vi "AcquireDataRamp.vi"(6 "error in":errorcluster, 11 "FPGA VI Reference In":T1) -> (2 "Elements Remaining":u32, 3 "FPGA VI Reference Out":T1, 4 "error out":errorcluster)   [LabVIEW 2016]
uses:
  controls/FPGAVIreferenceTypeDef.ctl
  controls/Enum.ctl
  <vilib>/Utility/error.llb/Error Cluster From Error Code.vi
  <vilib>/rvi/errors/niLvFpgaAdjustHostInterfaceError.vi
  <vilib>/rvi/interface/nirviMethod/nirviMethod.xnode
  FPGA Bitfiles/qnmController797_usbRIO_controllerFPGAmu_11012018-14h.lvbitx
  <vilib>/rvi/errors/niLvFpgaMergeErrorWithErrorCode.vi
  <vilib>/FPGAPlugInAG/USB-7856R OEM/niLvFpga_ReadFifo_USB-7856R OEM.vi
panel:
  # "Enable Error Handling disbaled (from VI properties)"
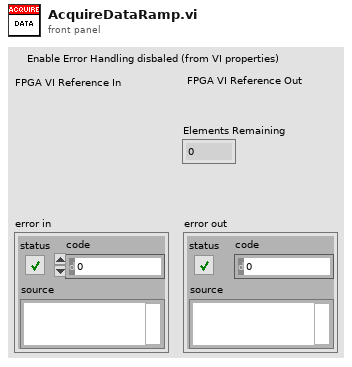
[diagram p1: front panel]
types:
  T1 = typedef "FPGAVIreferenceTypeDef.ctl" = refnum<k20>
  T2 = typedef "Enum.ctl" = enum16{"Init", "Read", "Write"}
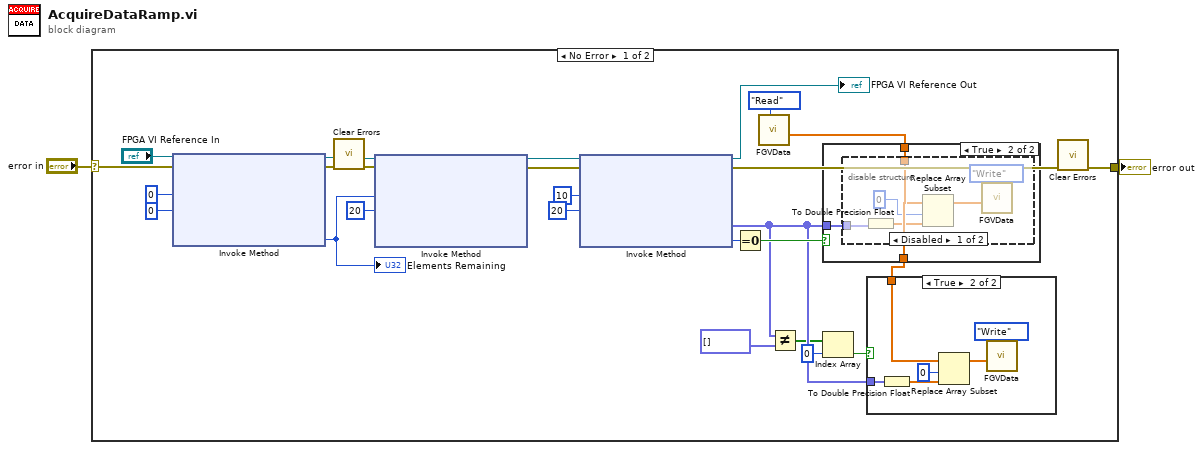
[diagram p0: block diagram]
diagram:
  n1 = case shown="No Error" "error in" {
    selector: "error in" -> [w16 w44]
    tunnel: [w22 w44] -> w2
    frame No Error {
      n2 = xnode "Invoke Method"("FPGA VI Reference In"="FPGA VI Reference In", "error in"=w16, "Number of Elements"=u32 0, "Timeout (ms)"=0) -> ("FPGA VI Reference Out"=w26:T1, "error out"=w28:errorcluster, "Elements Remaining"=w24:u32)  [unwired: 1 out]
      "Elements Remaining" <- w24
      n3 = call <vilib>:"Clear Errors.vi"("error in (no error)"=w28) -> ("error out"=w21:errorcluster)  [unwired: 5 in, 1 out]
      n4 = xnode "Invoke Method"("FPGA VI Reference In"=w26, "error in"=w21, "Number of Elements"=w24, "Timeout (ms)"=20) -> ("FPGA VI Reference Out"=w27:T1, "error out"=w20:errorcluster)  [unwired: 2 out]
      n5 = xnode "Invoke Method"("FPGA VI Reference In"=w27, "error in"=w20, "Number of Elements"=u32 10, "Timeout (ms)"=20) -> ("FPGA VI Reference Out"=→"FPGA VI Reference Out":T1, "error out"=w23:errorcluster, "Data"=w7:fxp<+/-,18,1>[], "Elements Remaining"=w11:u32)
      n6 = Equal To 0?(x=w11) -> (x = 0?=w10:bool)
      n7 = call "FGVData.vi"("Enum"=Enum."Read") -> ("DataOut"=w19:dbl[])  [unwired: 9 in, 1 out]
      n8 = Not Equal?(x=w7, y=fxp<+/-,18,1>[] [] ("Data")) -> (x != y?=w6:bool[])
      n9 = case shown="True" w10 {
        tunnel: w19 -> [w35 w36]
        tunnel: w7 -> [_ w37]
        tunnel: [w35 w36] -> w8
        frame False {
        }
        frame True {
          n10 = disable-structure shown="Disabled" {
            disable-tunnel: w37 -> [w40 _]
            disable-tunnel: w36 -> [w38 _]
            frame Disabled {
              n11 = To Double Precision Float(number=w40) -> (double precision float=w41:dbl[])
              n12 = Replace Array Subset(array=w38, new element=w41, index=0) -> (w43:dbl[])
              n13 = call "FGVData.vi"("Enum"=Enum."Write", "DataIn"=w43) -> ()  [unwired: 8 in, 2 out]
            }
            frame Enabled {
            }
          }
        }
      }
      n14 = Index Array(array=w6, index=0) -> (element=w4:bool)
      n15 = case shown="True" w4 {
        tunnel: w8 -> [_ w30]
        tunnel: w7 -> [_ w29]
        frame False {
        }
        frame True {
          n16 = To Double Precision Float(number=w29) -> (double precision float=w33:dbl[])
          n17 = Replace Array Subset(array=w30, new element=w33, index=0) -> (w31:dbl[])
          n18 = call "FGVData.vi"("Enum"=Enum."Write", "DataIn"=w31) -> ()  [unwired: 8 in, 2 out]
        }
      }
      n19 = call <vilib>:"Clear Errors.vi"("error in (no error)"=w23) -> ("error out"=w22:errorcluster)  [unwired: 5 in, 1 out]
    }
    frame Error {
    }
  }
  "error out" <- w2
